vi "hex parse.vi"() -> ()   [LabVIEW 2017]
panel:
  out "x/y":dbl
  out "number":i32
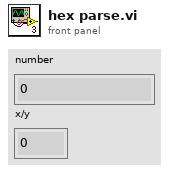
[diagram p1: front panel]
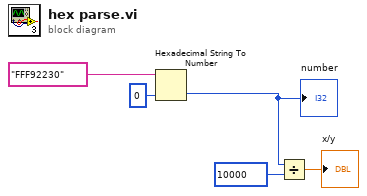
[diagram p0: block diagram]
diagram:
  n1 = Hexadecimal String To Number(string="FFF92230", default (0uL)=0 ("default (0 U32)")) -> (number=w3:i32)  [unwired: 1 in, 1 out]
  "number" <- w3
  n2 = Divide(x=w3, y=10000) -> (x/y=→"x/y":dbl)
